vi "ActionVIOnRecompile.vi"(8 "error in":errorcluster, 9 "Timeout (ms)":u32, 10 "node_path":string, 11 "Device Item Ref in":T1 format="%.0x") -> (0 "error out":errorcluster)   [LabVIEW 2025, in "Runtime Configuration Support Inline Async Example System Explorer.lvlib"]
uses:
  Runtime Configuration Support Inline Async Example System Explorer.lvlib
  <vilib>/NI VeriStand/Custom Device API/Custom Device Item Ref.ctl
  <vilib>/NI VeriStand/Custom Device API/Custom Device Channel Type.ctl
  Shared/ReConfigured.Settings.ctl
  Shared/Compiled.Settings.ctl
  <vilib>/NI VeriStand/Custom Device API/Block Data Reference.ctl
  <vilib>/NI VeriStand/Custom Device API/Data Reference.ctl
  <vilib>/NI VeriStand/Custom Device API/Get Item Property (I32).vi
  Error Constants.vi
  <vilib>/NI VeriStand/Custom Device API/Get Item Property (Variant).vi
  <vilib>/NI VeriStand/Execution/CustomDevice/NI VeriStand - Send Custom Device Message (Byte Array).vi
  <vilib>/NI VeriStand/Custom Device API/Custom Device API.lvlib
  <vilib>/NI VeriStand/execution/CustomDevice/NI_VS Custom Device ExecutionAPI.lvlib
  <vilib>/NI/NIVS Inline Async API/_Data Access System Explorer/Data Access System Explorer.lvlib
  Shared/Runtime Configuration Support Inline Async Example Shared.lvlib
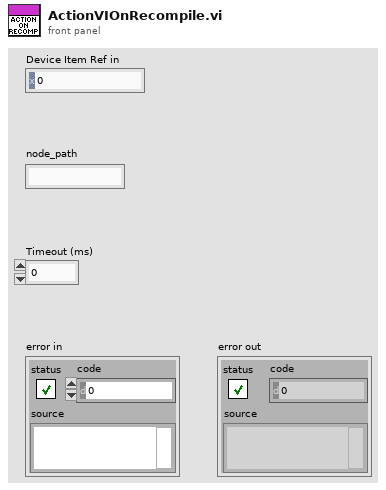
[diagram p1: front panel]
types:
  T1 = typedef "Custom Device API.lvlib/Custom Device Item Ref.ctl" = u64
  T2 = typedef "Runtime Configuration Support Inline Async Example Shared.lvlib/ReConfigured.Settings.ctl" = cluster{"Compiled.Settings":T3, "Compiled Inline Async Settings":cluster{"Read":cluster{"Refs":T4[], "Values":dbl[]}[], "Write":cluster{"Refs":T4[], "Values":dbl[]}[], "ReadWrite":cluster{"Refs":T5[], "Values":dbl[], "Reset Values":dbl[]}[], "LUT":variant}, "Response Ref":refnum<queue>}
  T3 = typedef "Runtime Configuration Support Inline Async Example Shared.lvlib/Compiled.Settings.ctl" = cluster{"Name":string, "Async Init Timeout":u16, "Inport SignalIDs":i32[], "Outport SignalIDs":i32[], "Inport Values":dbl[], "Outport Values":dbl[], "Dynamic Config Status":bool, "Device Error":errorcluster}
  T4 = typedef "Custom Device API.lvlib/Block Data Reference.ctl" = cluster{"Data Reference":T5, "Offset":u64, "Length":u64}
  T5 = typedef "Custom Device API.lvlib/Data Reference.ctl" = i32
  T6 = cluster{"Name":string, "Type":enum16{"Output/Write", "Input/Read", "Input/ReadWrite"}, "VS Refs":T1[]}
  T7 = enum16{"Output/Write", "Input/Read", "Input/ReadWrite"}
  T8 = cluster{"Dynamic Config Status":bool, "Error":errorcluster}
  T9 = typedef "Custom Device API.lvlib/Custom Device Channel Type.ctl" = enum16{"Input", "Output"}
  T10 = cluster{"Read":cluster{"Refs":T4[], "Values":dbl[]}[], "Write":cluster{"Refs":T4[], "Values":dbl[]}[], "ReadWrite":cluster{"Refs":T5[], "Values":dbl[], "Reset Values":dbl[]}[], "LUT":variant}
  T11 = cluster{"Name":string, "Type":enum16{"Output/Write", "Input/Read", "Input/ReadWrite"}, "VS Refs":T1[]}[]
  T12 = typedef "NI_VS Custom Device ExecutionAPI.lvlib/Custom Device Ref.ctl" = refnum<k24>
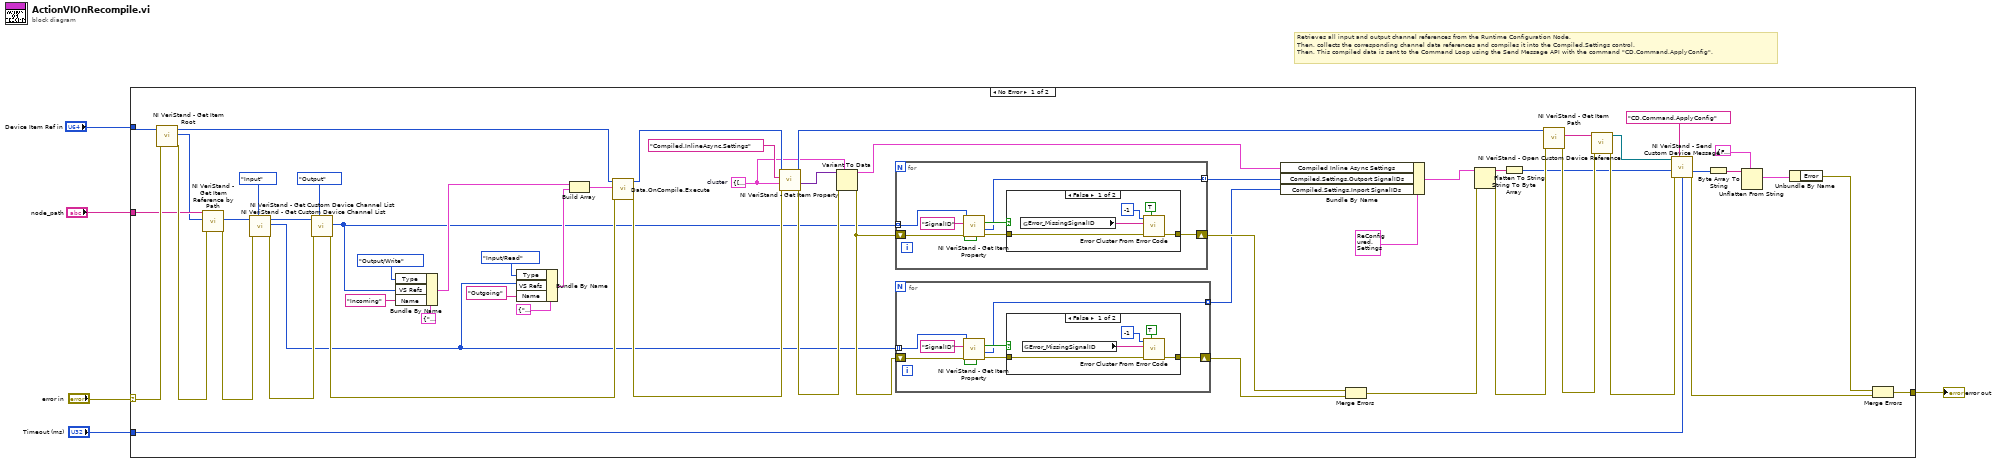
[diagram p0: block diagram]
diagram:
  # "Retrieves all input and output channel references from the Runtime Configuration Node.\nThen, collects the corresponding channel data references and compiles it into the Compiled.Settings control.\nThen, This compiled data is sent to the Command Loop using the Send Message API with the command \"CD.Command.ApplyConfig\"."
  n1 = case shown="No Error" "error in" {
    selector: "error in" -> [w54 w88]
    tunnel: [w49 w88] -> w4
    tunnel: "Device Item Ref in" -> [w39 _]
    tunnel: "node_path" -> [w40 _]
    tunnel: "Timeout (ms)" -> [w6 _]
    frame No Error {
      w8 = T10 {"Read"=[], "Write"=[], "ReadWrite"=[], "LUT"=variant}  # cluster
      n2 = call <vilib>:"NI VeriStand - Get Item Root.vi"("error in (no error)"=w54, "Item Ref in"=w39) -> ("error out"=w58:errorcluster, "Root Ref out"=w38:T1, "Item Ref out"=w17:T1)  [unwired: 6 in, 1 out]
      n3 = call <vilib>:"NI VeriStand - Get Item Reference by Path.vi"("error in (no error)"=w58, "Root Ref"=w38, "Item Path in"=w40) -> ("error out"=w57:errorcluster, "Item Ref"=w36:T1)  [unwired: 5 in, 2 out]
      n4 = call <vilib>:"NI VeriStand - Get Custom Device Channel List.vi"("Channel Type"=Custom_Device_Channel_Type."Input", "error in (no error)"=w57, "Device Ref in"=w36) -> ("error out"=w61:errorcluster, "Specified Channel Ref List"=w14:T1[], "Device Ref out"=w37:T1)  [unwired: 6 in]
      n5 = call <vilib>:"NI VeriStand - Get Custom Device Channel List.vi"("Channel Type"=Custom_Device_Channel_Type."Output", "error in (no error)"=w61, "Device Ref in"=w37) -> ("error out"=w48:errorcluster, "Specified Channel Ref List"=w15:T1[])  [unwired: 6 in, 1 out]
      n6 = Bundle By Name(cluster=T6 {"Name"="", "Type"=enum."Output/Write", "VS Refs"=[]} ("Group"), "Type"=T7."Output/Write", "VS Refs"=w15, "Name"="Incoming") -> (w20:T6)
      n7 = Bundle By Name(cluster=T6 {"Name"="", "Type"=enum."Output/Write", "VS Refs"=[]} ("Group"), "Type"=T7."Input/Read", "VS Refs"=w14, "Name"="Outgoing") -> (w19:T6)
      n8 = Build Array(w20, w19) -> (w18:T11)
      n9 = call <vilib>:"Data.OnCompile.Execute.vi"("error in"=w48, "VS Ref Groups"=w18, "Custom Device Ref"=w17) -> ("error out"=w46:errorcluster, "Custom Device Ref"=w12:T1)  [unwired: 6 in, 1 out]
      n10 = call-poly <vilib>:"NI VeriStand - Get Item Property.vi"("error in (no error)"=w46, "Default Value"=w8, "Property Name"="Compiled.InlineAsync.Settings", "Item Ref in"=w12) -> ("error out"=w47:errorcluster, "Value"=w9:variant, "Item Ref out"=w11:T1)  [unwired: 4 in, 1 out]
      n11 = Variant To Data(error in=w47, type=w8, Variant=w9) -> (data=w7:T10, error out=w45:errorcluster)
      n12 = for {
        tunnel: w15 -> [w65] mode=indexing
        shift-right: [w66] -> w55
        shift-left: w45 -> [w68]
        tunnel: [w62] -> w32 mode=indexing
        n13 = call-poly <vilib>:"NI VeriStand - Get Item Property.vi"("error in (no error)"=w68, "Property Name"="SignalID", "Item Ref in"=w65) -> ("error out"=w67:errorcluster, "Value"=w62:i32, "Found?"=w63:bool)  [unwired: 5 in, 1 out]
        n14 = case shown="False" w63 {
          tunnel: w67 -> [w73 w74]
          tunnel: [w72 w74] -> w66
          frame False {
            n15 = global read "Error Constants.vi" "Error_MissingSignalID"() -> (w69:string)
            n16 = call <vilib>:"Error Cluster From Error Code.vi"("show call chain? (False)"=TRUE, "error in (no error)"=w73, "error message (\"\")"=w69, "error code (0)"=-1) -> ("error out"=w72:errorcluster)  [unwired: 5 in]
          }
          frame True {
          }
        }
      }
      n17 = for {
        tunnel: w14 -> [w78] mode=indexing
        shift-right: [w79] -> w53
        shift-left: w45 -> [w81]
        tunnel: [w75] -> w30 mode=indexing
        n18 = call-poly <vilib>:"NI VeriStand - Get Item Property.vi"("error in (no error)"=w81, "Property Name"="SignalID", "Item Ref in"=w78) -> ("error out"=w80:errorcluster, "Value"=w75:i32, "Found?"=w76:bool)  [unwired: 5 in, 1 out]
        n19 = case shown="False" w76 {
          tunnel: w80 -> [w86 w87]
          tunnel: [w85 w87] -> w79
          frame False {
            n20 = global read "Error Constants.vi" "Error_MissingSignalID"() -> (w82:string)
            n21 = call <vilib>:"Error Cluster From Error Code.vi"("show call chain? (False)"=TRUE, "error in (no error)"=w86, "error message (\"\")"=w82, "error code (0)"=-1) -> ("error out"=w85:errorcluster)  [unwired: 5 in]
          }
          frame True {
          }
        }
      }
      n22 = Bundle By Name(cluster=T2 {"Compiled.Settings"={"Name"="", "Async Init Timeout"=0, "Inport SignalIDs"=[], "Outport SignalIDs"=[], "Inport Values"=[], "Outport Values"=[], "Dynamic Config Status"=FALSE, "Device Error"={"status"=FALSE, "code"=0, "source"=""}}, "Compiled Inline Async Settings"={"Read"=[], "Write"=[], "ReadWrite"=[], "LUT"=variant}, "Response Ref"=refnum} ("ReConfigured.Settings"), "Compiled Inline Async Settings"=w7, "Compiled.Settings.Outport SignalIDs"=w32, "Compiled.Settings.Inport SignalIDs"=w30) -> (w31:T2)
      n23 = Merge Errors(w55, w53) -> (w52:errorcluster)
      n24 = Flatten To String(anything=w31, error in (no error)=w52) -> (data string=w34:string, error out=w60:errorcluster)  [unwired: 2 in, 1 out]
      n25 = String To Byte Array(string=w34) -> (unsigned byte array=w33:u8[])
      n26 = call <vilib>:"NI VeriStand - Get Item Path.vi"("error in (no error)"=w60, "Item Ref in"=w11) -> ("error out"=w59:errorcluster, "Path"=w41:string)  [unwired: 6 in, 2 out]
      n27 = call <vilib>:"NI VeriStand - Open Custom Device Reference.vi"("error in (no error)"=w59, "Custom Device Path"=w41) -> ("error out"=w56:errorcluster, "Custom Device"=w35:T12)  [unwired: 8 in]
      n28 = call-poly <vilib>:"NI VeriStand - Send Custom Device Message.vi"("Timeout ms (5000)"=w6, "error in (no error)"=w56, "Data"=w33, "Command"="CD.Command.ApplyConfig", "Custom Device in"=w35) -> ("error out"=w51:errorcluster, "Response"=w29:u8[])  [unwired: 4 in, 1 out]
      n29 = Byte Array To String(unsigned byte array=w29) -> (string=w28:string)
      n30 = Unflatten From String(type=T8 {"Dynamic Config Status"=FALSE, "Error"={"status"=FALSE, "code"=0, "source"=""}}, binary string=w28) -> (value=w27:T8)  [unwired: 3 in, 2 out]
      n31 = Unbundle By Name(w27) -> ("Error"=w50:errorcluster)
      n32 = Merge Errors(w50, w51) -> (w49:errorcluster)
    }
    frame Error {
    }
  }
  "error out" <- w4
